vi "SCAN_VISA.vi"(8 "errin":errorcluster) -> (0 "sortie d'erreur":errorcluster, 3 "Refnum VISA en sortie":refnum<visa-resource-name>)   [LabVIEW 2020]
uses:
  <vilib>/Instr/_visa.llb/VISA Find Search Mode.ctl
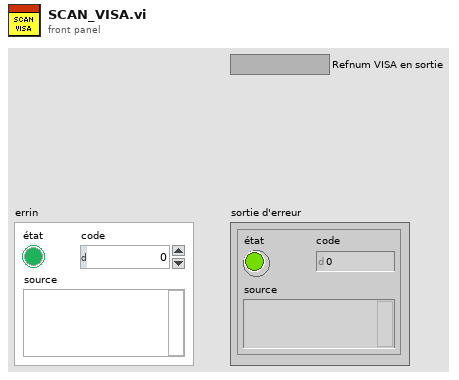
[diagram p1: front panel]
types:
  T1 = typedef "VISA Find Search Mode.ctl" = u32
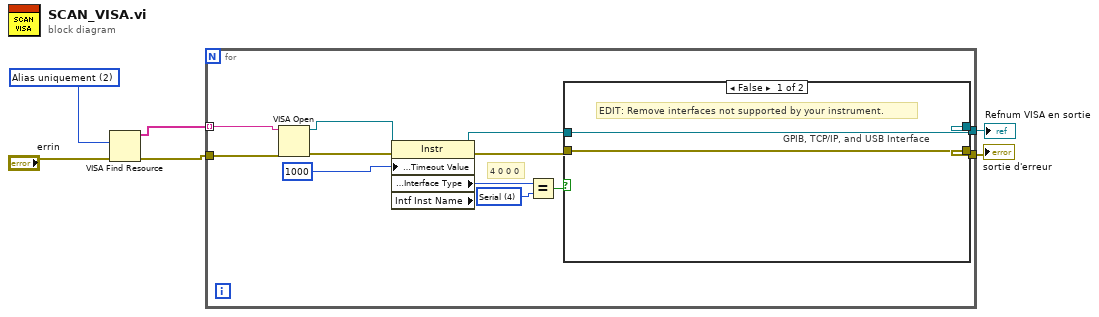
[diagram p0: block diagram]
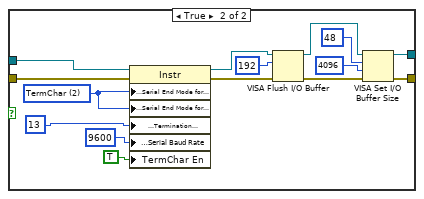
[diagram p2: hidden frame]
diagram:
  w2 = T1 2 items=["Noms canoniques uniquement"=0, "Alias uniquement"=2, "Inclure les alias correspondants"=3, "Inclure tous les alias"=4] ("Search Mode")
  n1 = VISA Find Resource(8:"errin", 10:w2) -> (0:w4:errorcluster, 3:w1:string[])  [unwired: 1 in, 1 out]
  n2 = for {
    tunnel: w4 -> [w12]
    tunnel: [w11] -> w5
    tunnel: [w10] -> w6
    tunnel: w1 -> [w7] mode=indexing
    w17 = u16 4 items=["GPIB"=1, "VXI"=2, "GPIB-VXI"=3, "Serial"=4, "PXI"=5, "TCPIP"=6, "USB"=7] ("Interface Information:Interface Type")
    # "4 0 0 0"
    n3 = VISA Open(error in (no error)=w12, VISA resource name=w7) -> (VISA resource name=w9:refnum<visa-resource-name>, error out=w8:errorcluster)  [unwired: 3 in]
    n4 = property class="Instr" props=["General Settings:Timeout Value", "Interface Information:Interface Type", "Intf Inst Name"](reference=w9, error in=w8, "General Settings:Timeout Value"=u32 1000) -> (reference out=w14:refnum<visa-resource-name>, error out=w13:errorcluster, "Interface Information:Interface Type"=w16:u16)  [unwired: 1 out]
    n5 = Equal?(x=w16, y=w17) -> (x = y?=w15:bool)
    n6 = case shown="False" w15 {
      tunnel: [w19 w22] -> w11
      tunnel: [w20 w23] -> w10
      tunnel: w14 -> [w19 w34]
      tunnel: w13 -> [w20 w35]
      frame False {
        # "EDIT: Remove interfaces not supported by your instrument."
        # "GPIB, TCP/IP, and USB Interface"
      }
      frame True {
        w26 = u16 2 items=["None", "LastBit", "TermChar"] ("Serial Settings:Serial End Mode for Reads")
        n7 = property class="Instr"(reference=w34, error in=w35, "Serial Settings:Serial End Mode for Reads"=w26, "Serial Settings:Serial End Mode for Writes"=w26, "Message Based Settings:Termination Character"=u8 13, "Serial Settings:Serial Baud Rate"=u32 9600 ("Serial Settings:Baud Rate"), "TermChar En"=TRUE ("Message Based Settings:Termination Character Enable")) -> (reference out=w30:refnum<visa-resource-name>, error out=w32:errorcluster)
        n8 = VISA Flush I/O Buffer(VISA resource name=w30, mask (16)=u16 192, error in (no error)=w32) -> (VISA resource name out=w33:refnum<visa-resource-name>, error out=w31:errorcluster)
        n9 = VISA Set I/O Buffer Size(VISA resource name=w33, mask (16)=u16 48, size (4096)=u32 4096 ("size (0)"), error in (no error)=w31) -> (VISA resource name out=w22:refnum<visa-resource-name>, error out=w23:errorcluster)
      }
    }
  }
  "Refnum VISA en sortie" <- w5
  "sortie d'erreur" <- w6
